vi "Execute.vi"(8 "error in":errorcluster, 9 "Consumer Queues in":T1, 10 "DAC Process Command in":refnum<class "Setup DAC Test Stand.lvclass">, 11 "DAC Process Data in":T2) -> (0 "error out":errorcluster, 1 "Consumer Queues out":T1, 2 "Stop?":bool, 3 "DAC Process Data out":T2)   [LabVIEW 2019, in "DAC Process.lvlib" / "Setup DAC Test Stand.lvclass"]
uses:
  Setup DAC Test Stand.lvclass
  DAC Process Data.ctl
  Generic Test Stand/Generic Test Stand.lvclass
  TS Framework/ExeLogging/DAC Logger/DAC Logger.lvclass
  DAC State.ctl
  TS Framework/Consumer Queues.ctl
  UI Process/Generic UI Command/Generic UI Process Command.lvclass
  Generic DAC Command/Generic DAC Process Command.lvclass
  Trig Process/Generic Trig Command/Generic Trig Process Command.lvclass
  Configure DAC Front Panel/Configure DAC Front Panel.lvclass
  UI Process/Update UI Status/Update UI Status.lvclass
  Setup DAC Test Stand.lvclass/Setup DAC Test Stand.ctl
  UI Process/Update UI Status/Update UI Status.lvclass/Update UI Status.ctl
  DAC Process.lvlib
  TS Framework/TS Framework.lvlib
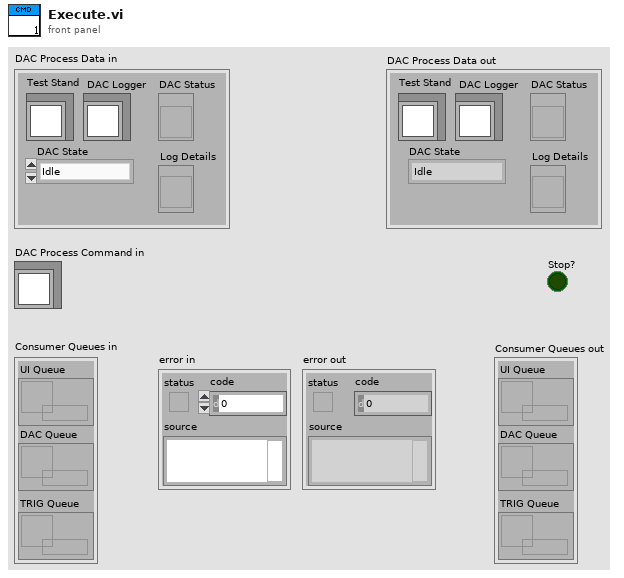
[diagram p1: front panel]
types:
  T1 = typedef "TS Framework.lvlib/Consumer Queues.ctl" = cluster{"UI Queue":refnum<queue>, "DAC Queue":refnum<queue>, "TRIG Queue":refnum<queue>}
  T2 = typedef "DAC Process.lvlib/DAC Process Data.ctl" = cluster{"Test Stand":refnum<class "Generic Test Stand.lvclass">, " DAC Logger":refnum<class "DAC Logger.lvclass">, "DAC State":T3, "DAC Status":refnum<vi>, "Log Details":refnum<vi>}
  T3 = typedef "DAC Process.lvlib/DAC State.ctl" = enum16{"Idle", "Acquiring"}
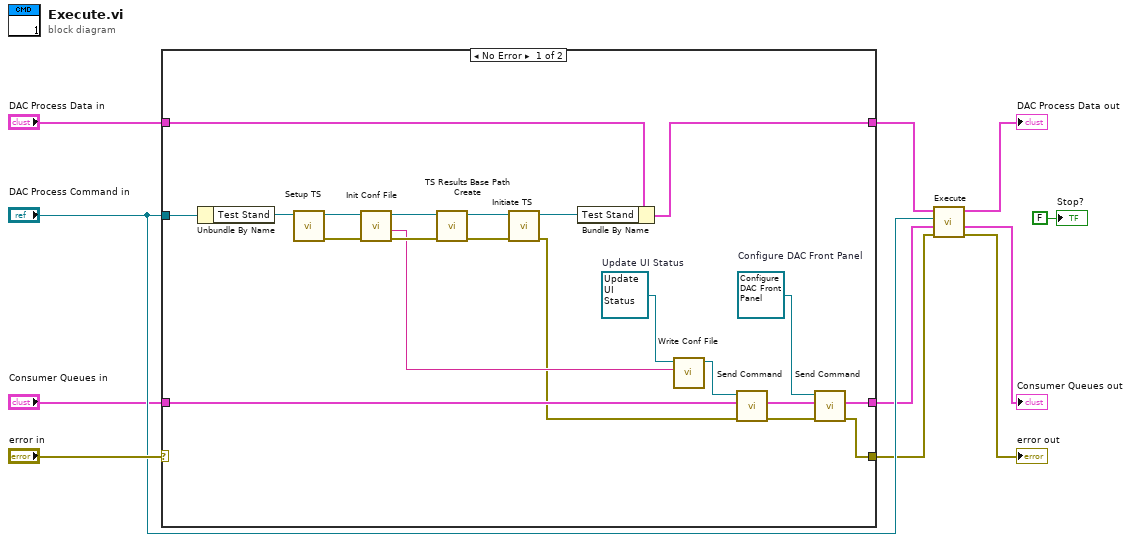
[diagram p0: block diagram]
diagram:
  n1 = case shown="No Error" "error in" {
    selector: "error in" -> [_ w35]
    tunnel: "DAC Process Command in" -> [w32 _]
    tunnel: "DAC Process Data in" -> [w30 w33]
    tunnel: "Consumer Queues in" -> [w25 w34]
    tunnel: [w26 w35] -> w3
    tunnel: [w28 w34] -> w2
    tunnel: [w29 w33] -> w4
    frame No Error {
      w22 = refnum<class "Update UI Status.lvclass"> refnum  # Update UI Status
      w27 = refnum<class "Configure DAC Front Panel.lvclass"> refnum  # Configure DAC Front Panel
      n2 = Unbundle By Name(w32) -> ("Test Stand"=w31:refnum<class "Generic Test Stand.lvclass">)
      n3 = call-dynamic "Setup TS.vi"("Generic Test Stand in"=w31) -> ("error out"=w18:errorcluster, "Generic Test Stand out"=w20:refnum<class "Generic Test Stand.lvclass">)  [unwired: 9 in]
      n4 = call "Init Conf File.vi"("error in"=w18, "Test Stand in"=w20) -> ("error out"=w17:errorcluster, "Conf Filename"=w16:string, "Test Stand out"=w19:refnum<class "Generic Test Stand.lvclass">)  [unwired: 7 in]
      n5 = call-dynamic "TS Results Base Path Create.vi"("error in"=w17, "Generic Test Stand in"=w19) -> ("error out"=w14:errorcluster, "Generic Test Stand out"=w15:refnum<class "Generic Test Stand.lvclass">)  [unwired: 8 in]
      n6 = call-dynamic "Initiate TS.vi"("error in (no error)"=w14, "Generic Test Stand in"=w15) -> ("error out"=w12:errorcluster, "Generic Test Stand out"=w13:refnum<class "Generic Test Stand.lvclass">)  [unwired: 8 in]
      n7 = Bundle By Name(cluster=w30, "Test Stand"=w13) -> (w29:T2)
      n8 = call "Write Conf File.vi"("Conf File"=w16, "Update UI Status in"=w22) -> ("Update UI Status out"=w23:refnum<class "Update UI Status.lvclass">)  [unwired: 9 in]
      n9 = call-dynamic "Send Command.vi"("error in (no error)"=w12, "Consumer Queues in"=w25, "UI Process Command in"=w23) -> ("error out"=w21:errorcluster, "Consumer Queues out"=w24:T1)  [unwired: 7 in]
      n10 = call-dynamic "Send Command.vi"("error in (no error)"=w21, "Consumer Queues in"=w24, "DAC Process Command"=w27) -> ("error out"=w26:errorcluster, "Consumer Queues out"=w28:T1)  [unwired: 7 in]
    }
    frame Error {
    }
  }
  n11 = call-parent "Execute.vi"("error in"=w3, "Consumer Queues in"=w2, "DAC Process Command in"="DAC Process Command in", "DAC Process Data in"=w4) -> ("error out"=→"error out":errorcluster, "Consumer Queues out"=→"Consumer Queues out":T1, "DAC Process Data out"=→"DAC Process Data out":T2)  [unwired: 4 in, 1 out]
  "Stop?" <- FALSE ("Stop?")
